vi "GET_UserLayers.vi"(8 "error in (no error)":errorcluster, 11 "Icon.lvclass in":refnum<class "Icon.lvclass">) -> (0 "error out":errorcluster, 1 "Active Layer":refnum<class "Layer.lvclass">, 2 "All Layers":refnum<class "Layer.lvclass">[](array[class]), 3 "Icon.lvclass out":refnum<class "Icon.lvclass">, 4 "#Active Layer":i32, 6 "Layer Locked?":bool)   [LabVIEW 2017, in "Icon.lvclass"]
doc: "Returns all User Layers, as well as the active User Layer, its index and whether or not it is locked."
uses:
  <vilib>/LabVIEW Icon API/lv_icon/Classes/Icon/Icon.lvclass
  <vilib>/LabVIEW Icon API/lv_icon/Classes/Layer/Layer.lvclass
  <vilib>/LabVIEW Icon API/lv_icon/Classes/Icon/Icon.lvclass/Icon.ctl
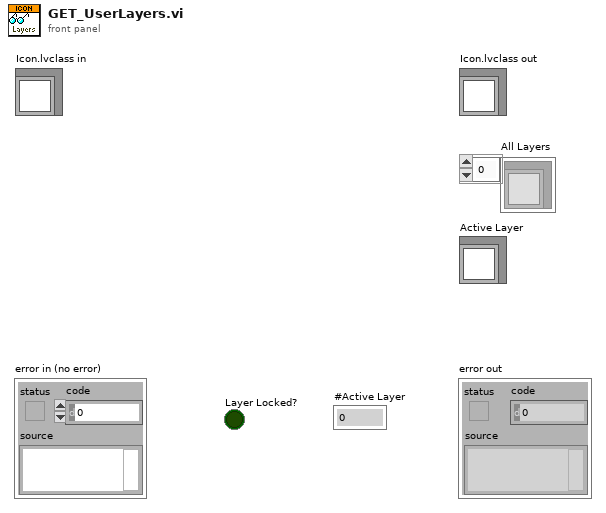
[diagram p1: front panel]
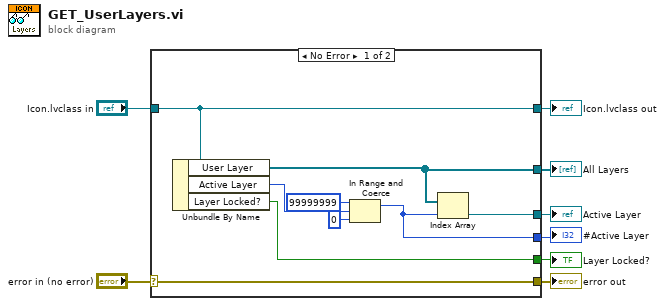
[diagram p0: block diagram]
diagram:
  n1 = case shown="No Error" "error in (no error)" {
    selector: "error in (no error)" -> [w17 w18]
    tunnel: [w17 w18] -> w7
    tunnel: [w16 w19] -> w5
    tunnel: "Icon.lvclass in" -> [w16 w19]
    tunnel: [w15 _] -> w4
    tunnel: [w14 _] -> w3
    tunnel: [w9 _] -> w2
    tunnel: [w13 _] -> w1
    frame No Error {
      n2 = Unbundle By Name(w16) -> ("User Layer"=w15:refnum<class "Layer.lvclass">[], "Active Layer"=w10:i32, "Layer Locked?"=w13:bool)
      n3 = In Range and Coerce(upper limit=99999999, x=w10, lower limit=0) -> (coerced(x)=w9:i32)  [unwired: 1 out]
      n4 = Index Array(array=w15, index=w9) -> (element=w14:refnum<class "Layer.lvclass">)
    }
    frame Error {
    }
  }
  "error out" <- w7
  "Icon.lvclass out" <- w5
  "All Layers" <- w4
  "Active Layer" <- w3
  "#Active Layer" <- w2
  "Layer Locked?" <- w1
